vi "Exercice4-2.vi"() -> ()   [LabVIEW 2013]
panel:
  in  "Bouton rotatif":dbl(knob) scale=0.0..2.0
  out "Historique":dbl(graph)
  in  "Stop":bool=TRUE
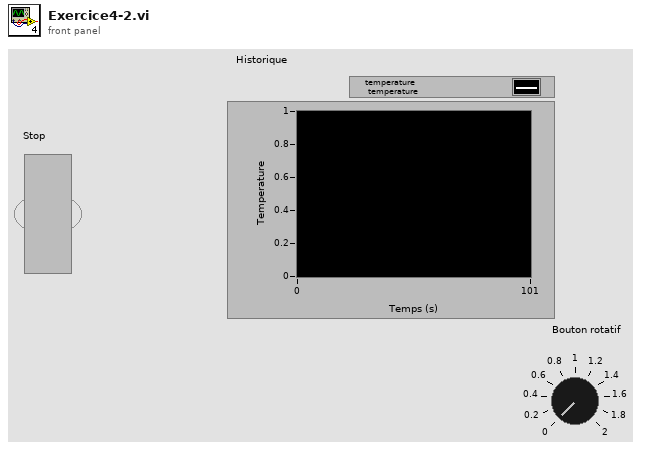
[diagram p1: front panel]
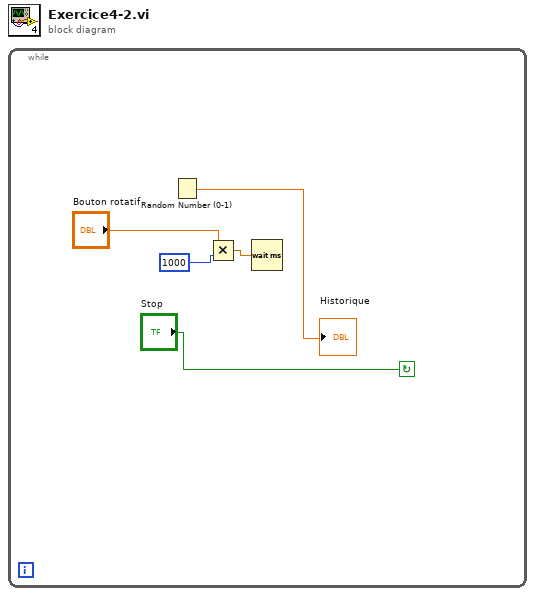
[diagram p0: block diagram]
diagram:
  n1 = while {
    stop <- "Stop" continue-if-true
    n2 = Random Number (0-1)() -> (number: 0 to 1=→"Historique":dbl)
    n3 = Multiply(x="Bouton rotatif", y=1000) -> (x*y=w3:dbl)
    n4 = Wait (ms)(milliseconds to wait=w3) -> ()  [unwired: 1 out]
  }
